vi "TB-Choose Slack User Dialog.vi"(0 "users":T1[](array[typedef]), 2 "CtlRef":refnum<vi>) -> (4 "users":cluster{"id":string, "always":bool}[](array[cluster]))   [LabVIEW 2020]
uses:
  Typedefs/TB-User.ctl
panel:
  out "Listbox":i32(listbox) caption="Choose Slack recipients"
  in  "OK":bool
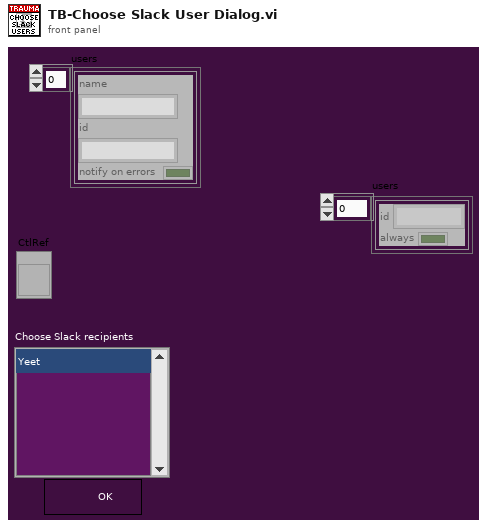
[diagram p1: front panel]
types:
  T1 = typedef "TB-User.ctl" = cluster{"name":string, "id":string, "notify on errors":bool}
  T2 = cluster{"id":string, "notify on errors":bool, bool}
  T3 = cluster{"Left":i16, "Top":i16, "Right":i16, "Bottom":i16, "Width":i16, "Height":i16}
  T4 = cluster{"id":string, "notify on errors":bool, bool}[]
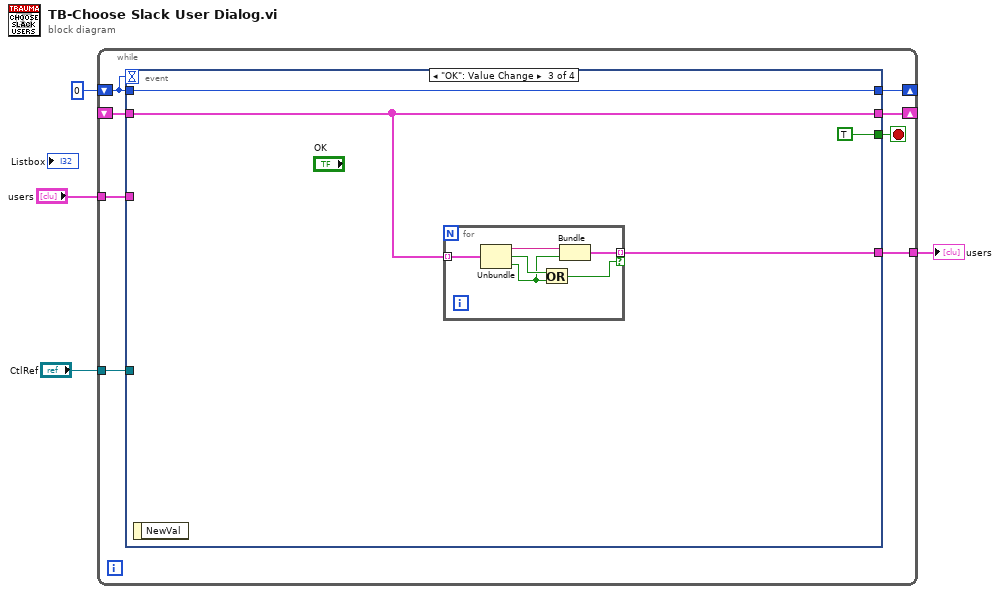
[diagram p0: block diagram]
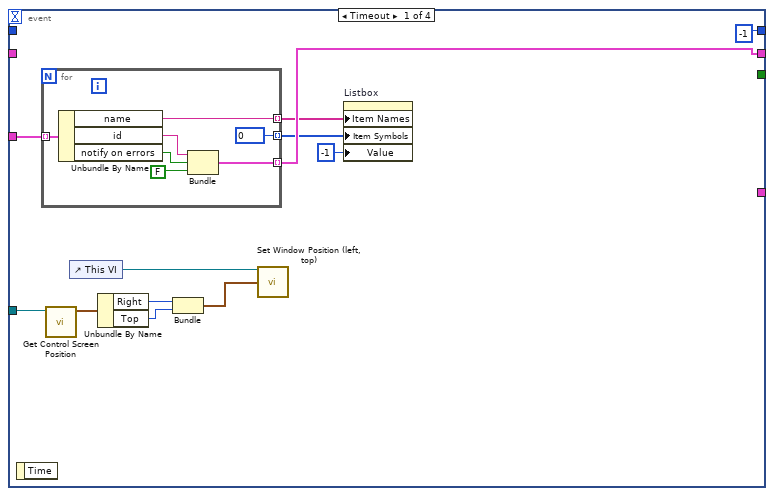
[diagram p2: hidden frame]
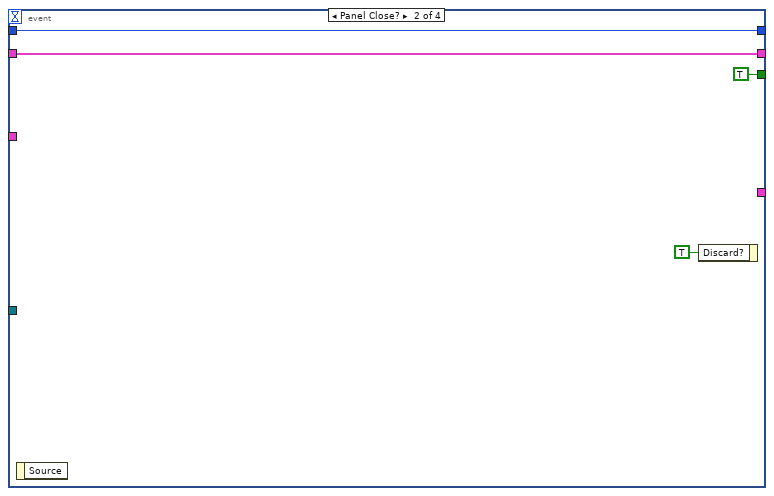
[diagram p3: hidden frame]
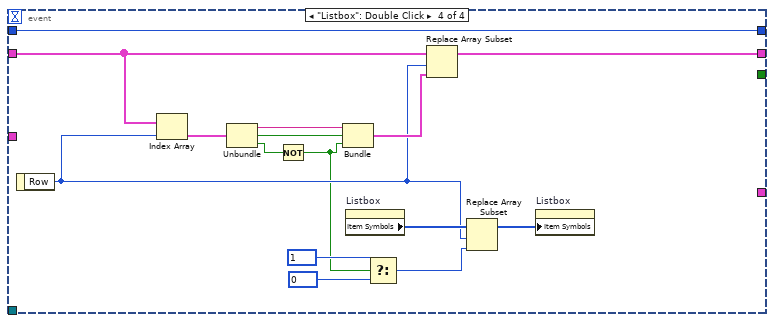
[diagram p4: hidden frame]
diagram:
  n1 = while {
    shift-right: [w12] -> _
    shift-left: 0 -> [w10]
    tunnel: "users" -> [w9]
    tunnel: "CtlRef" -> [w8]
    shift-right: [w7] -> _
    shift-left: _ -> [w6]
    tunnel: [w5] -> w1
    stop <- w11 stop-if-true
    n2 = event shown="[2] \"OK\": Value Change" {
      selector: _ -> [_ _ _ _]
      dyn-events: _ -> [_ _ _ _]
      timeout: w10 -> [_ _ _ _]
      tunnel: [-1 w35 w38 w60] -> w12
      tunnel: [_ TRUE TRUE _] -> w11
      tunnel: w10 -> [_ w35 w38 w60]
      tunnel: w9 -> [w21 _ _ _]
      tunnel: w8 -> [w20 _ _ _]
      tunnel: [w15 w33 w37 w56] -> w7
      tunnel: w6 -> [_ w33 w37 w57]
      tunnel: [_ _ w36 _] -> w5
      event Timeout {
        n3 = event-data() -> ()  [unwired: 1 in, 1 out]
        n4 = for {
          tunnel: w21 -> [w31] mode=indexing
          tunnel: [w29] -> w15 mode=indexing
          tunnel: [w26] -> w14 mode=indexing
          tunnel: [0] -> w13 mode=indexing
          n5 = Unbundle By Name(w31) -> ("name"=w26:string, "id"=w30:string, "notify on errors"=w27:bool)
          n6 = Bundle("id"=w30, "notify on errors"=w27, FALSE) -> (w29:T2)  [unwired: 1 in]
        }
        n7 = call "Get Control Screen Position.vi"("Control in"=w20) -> ("Bounds Out"=w19:T3)  [unwired: 10 in]
        n8 = control-ref of="This VI"() -> (w23:refnum<vi>)
        n9 = Unbundle By Name(w19) -> ("Right"=w17:i16, "Top"=w18:i16)
        n10 = Bundle("Right"=w17, "Top"=w18) -> (w22:cluster{"Right":i16, "Top":i16})  [unwired: 1 in]
        n11 = call "Set Window Position (left, top).vi"("VI in"=w23, "Coords"=w22) -> ()  [unwired: 12 in, 2 out]
        n12 = property on="Listbox" class="LstBox (strict)"("Item Names"=w14, "Item Symbols"=w13, "Value"=-1 ("Listbox")) -> ()  [unwired: 2 in, 2 out]
      }
      event Panel Close? {
        n13 = event-data() -> ()  [unwired: 1 in, 1 out]
        n14 = event-data("Discard?"=TRUE) -> ()  [unwired: 1 in, 1 out]
      }
      event "OK": Value Change {
        n15 = event-data() -> ()  [unwired: 1 in, 1 out]
        n16 = for {
          tunnel: w37 -> [w45] mode=indexing
          tunnel: [w41] -> w36 mode=indexing if=w44
          n17 = Unbundle(w45) -> ("id"=w43:string, "notify on errors"=w42:bool, w40:bool)
          n18 = Or(x=w42, y=w40) -> (x .or. y?=w44:bool)
          n19 = Bundle("id"=w43, w40) -> (w41:cluster{"id":string, bool})  [unwired: 1 in]
        }
      }
      event "Listbox": Double Click {
        n20 = event-data() -> ("Row"=w51:i32)  [unwired: 1 in]
        n21 = Index Array(array=w57, index=w51) -> (element=w59:T2)
        n22 = Unbundle(w59) -> ("id"=w58:string, "notify on errors"=w46:bool, w48:bool)
        n23 = Not(x=w48) -> (.not. x?=w47:bool)
        n24 = Bundle("id"=w58, "notify on errors"=w46, w47) -> (w55:T2)  [unwired: 1 in]
        n25 = property on="Listbox" class="LstBox (strict)"() -> ("Item Symbols"=w52:i32[])  [unwired: 2 in, 2 out]
        n26 = Select(t=1, s=w47, f=0) -> (s? t:f=w50:i32)
        n27 = Replace Array Subset(array=w57, new element=w55, index=w51) -> (w56:T4)
        n28 = Replace Array Subset(array=w52, new element=w50, index=w51) -> (w49:i32[])
        n29 = property on="Listbox" class="LstBox (strict)"("Item Symbols"=w49) -> ()  [unwired: 2 in, 2 out]
      }
    }
  }
  "users" <- w1
